vi "UTIL Piezo Feat.vi"(4 "init/cont (init:F)":bool, 7 "Piezo In":waveform(dbl)) -> (1 "Piezo Power":dbl format="%0.2f", 3 "Filtered Piezo Out":waveform(dbl))   [LabVIEW 2010]
doc: "This VI computed the r.m.s. power in the Piezo signal to serve as a surrogate fo EMG power in the task of sleep wake differentiation.\n\nInputs\n Piezo In Waveform\nOutputs\n Piezo Power DBL"
uses:
  <vilib>/Analysis/3filter.llb/IIR Filter (DBL).vi
  <vilib>/Analysis/NI_AALBase.lvlib
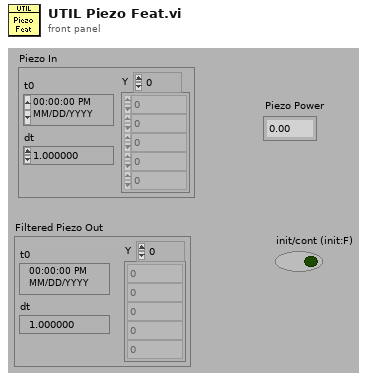
[diagram p1: front panel]
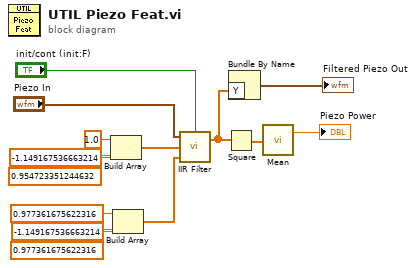
[diagram p0: block diagram]
diagram:
  n1 = Build Array(1.0 ("element"), -1.149167536663214 ("element"), 0.954723351244632 ("element")) -> (w6:dbl[])
  n2 = Build Array(0.977361675622316 ("element"), -1.149167536663214 ("element"), 0.977361675622316 ("element")) -> (w5:dbl[])
  n3 = call-poly <vilib>:"IIR Filter.vi"("init/cont (init:F)"="init/cont (init:F)", "Forward Coefficients"=w5, "Reverse Coefficients"=w6, "X"="Piezo In") -> ("Filtered X"=w2:dbl[])  [unwired: 1 out]
  n4 = Square(x=w2) -> (x^2=w14:dbl[])
  n5 = Bundle By Name("Y"=w2) -> (→"Filtered Piezo Out":waveform(dbl))  [unwired: 1 in]
  n6 = call <vilib>:"Mean.vi"("X"=w14) -> ("mean"=→"Piezo Power":dbl)  [unwired: 1 out]
